vi "CenterFinder_6points_2points.vi"() -> ()   [LabVIEW 2016]
uses:
  Control/ProcessCtl.ctl
  <vilib>/userdefined/High Color/IMAQdx.ctl
  <vilib>/Utility/config.llb/Read Key (String).vi
  <vilib>/Utility/config.llb/Write Key (Double).vi
  <vilib>/vision/driver/NI_Vision_Acquisition_Software.lvlib
  <vilib>/vision/NI_Vision_Development_Module.lvlib
  <vilib>/Utility/config.llb/NI_LVConfig.lvlib
panel:
  out "output cluster":T1
  out "Array":T2(array[cluster])
  in  "stop 2":bool
  out "1":u32[](array[colorbox])
  in  "MoveTo":bool
  out "Boolean":bool=TRUE
  in  "GoToXY":bool
  out "Tip Center":cluster{"X":dbl, "Y":dbl, "Z":dbl}
  in  "Minimum Edge Strength":dbl=10.0
  out "Camera Center":cluster{"X":dbl, "Y":dbl, "Z":dbl}
  in  "Delete":bool caption="Retake"
  in  "Retake":bool caption="Delete"
  in  "Next":bool
  in  "Process":bool
  in  "Acquire":bool
  in  "stop":bool
  out "Image":T3(plugin-control)
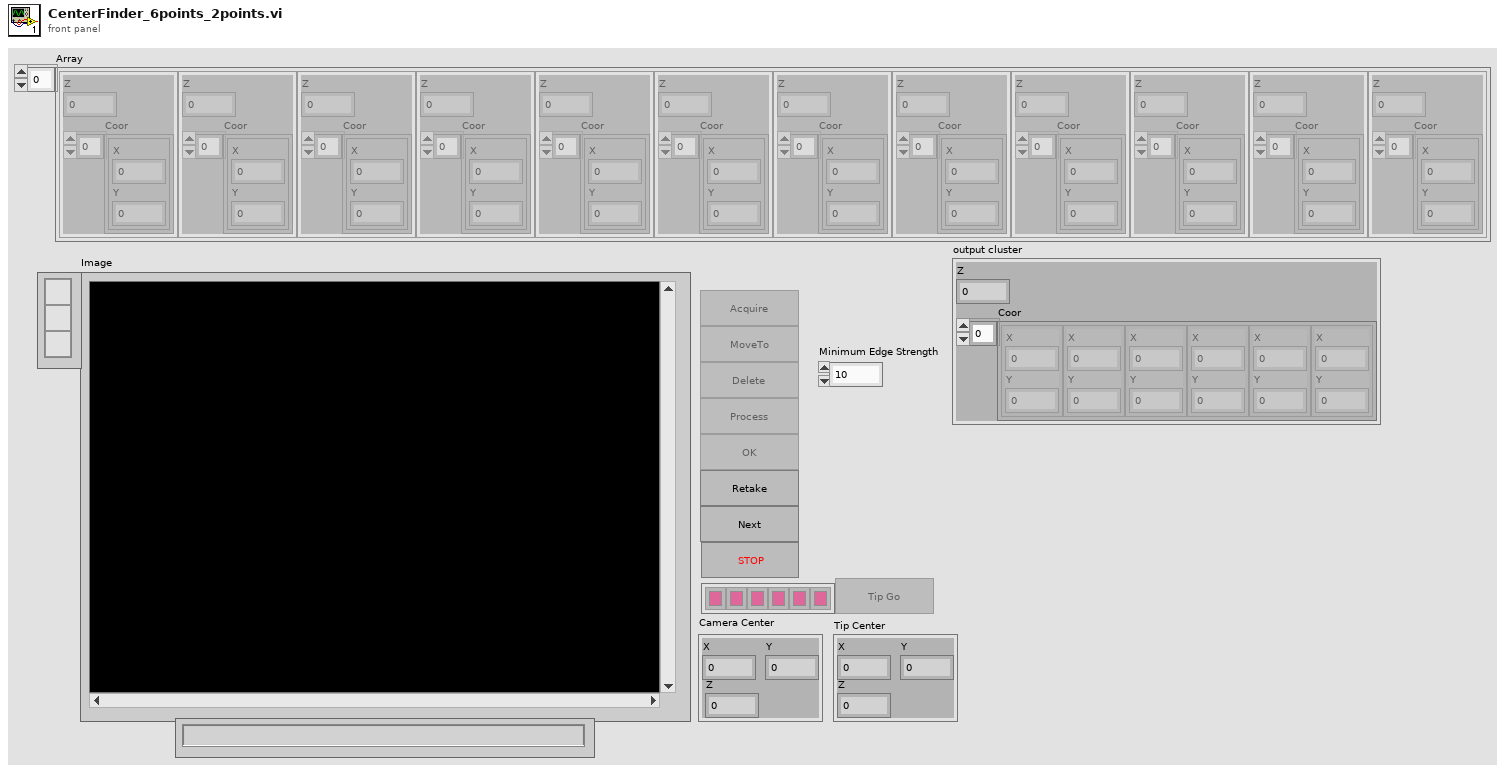
[diagram p1: front panel]
types:
  T1 = cluster{"Z":dbl, "Coor":cluster{"X":sgl, "Y":sgl}[]}
  T2 = cluster{"Z":dbl, "Coor":cluster{"X":sgl, "Y":sgl}[]}[]
  T3 = typedef "IMAQ Image.ctl" = refnum<image>
  T4 = cluster{"Line Segment":cluster{"Point 1":cluster{"X":sgl, "Y":sgl}, "Point 2":cluster{"X":sgl, "Y":sgl}}, "Z":dbl}[]
  T5 = typedef "IMAQdx.ctl" = refnum<k21>
  T6 = typedef "ProcessCtl.ctl" = enum16{"Idle", "Acquire", "Process", "Abort", "Initialize", "Wait"}
  T7 = typedef "NI_LVConfig.lvlib/Config Data RefNum.ctl" = refnum<k1>
  T8 = enum8{"Enabled", "Disabled", "Disabled and Grayed Out"}
  T9 = cluster{"Edge Polarity":u16, "Kernel Size":u32, "Width":u32, "Minimum Edge Strength":dbl, "Interpolation Type":u16, "Data Processing Method":u16}
  T10 = typedef "IMAQ Line" = cluster{"Start X":i32, "Start Y":i32, "End X":i32, "End Y":i32}
  T11 = typedef "Image Type" = u32
  T12 = typedef "ROI Descriptor" = cluster{"Global Rectangle":i32[], "Contours":cluster{"ID":enum32{"External", "Internal"}, "Type":u32, "Coordinates":i32[]}[]}
  T13 = cluster{"Global Rectangle":i32[], "Contours":cluster{"Contour Type":u32, "ROI Type":u32, "Points":i32[]}[]}
  T14 = typedef "Edge New.ctl" = cluster{"Location (Pixel)":cluster{"X":sgl, "Y":sgl}, "Location (Real-World)":cluster{"X":sgl, "Y":sgl}, "Distance (Pixel)":dbl, "Distance (Real-World)":dbl, "Strength":dbl, "Noise":dbl, "Rising?":bool}
  T15 = typedef "ControllerDiagPacket.ctl" = cluster{"Number of Diag Packets":i32, "Axes":T16[], "error":errorcluster}
  T16 = typedef "AxisDiagPacket.ctl" = cluster{"Axis Name":string, "Analog Input 0":dbl, "Analog Input 1":dbl, "Axis Fault (num)":i32, "Axis Fault (str)":string, "Axis Fault (bits)":cluster{"AmplifierFault":bool, "AmplifierTemperatureFault":bool, "CcwEndOfTravelLimitFault":bool, "CcwSoftwareLimitFault":bool, "CommunicationLostFault":bool, "CwEndOfTravelLimitFault":bool, "CwSoftwareLimitFault":bool, "EmergencyStopFault":bool, "EncoderFault":bool, "ExternalFault":bool, "FeedbackScalingFault":bool, "GantryMisalignFault ":bool, "HallSensorFault":bool, "InPositionTimeoutFault":bool, "InternalFault":bool, "MarkerSearchFault":bool, "MaxVelocityCommandFault":bool, "MissedInterruptFault":bool, "MotorTemperatureFault":bool, "None":bool, "OverCurrentFault":bool, "PositionErrorFault":bool, "PositionFeedbackFault":bool, "PowerSupplyFault":bool, "ProbeInputFault":bool, "SafeZoneFault":bool, "VelocityErrorFault":bool, "VelocityFeedbackFault":bool, "VoltageClampFault":bool}, "Axis Status (num)":i32, "Axis Status (str)":string, "Axis Status (bits)":cluster{"BacklashActive":bool, "CalibrationEnabled1D":bool, "CalibrationEnabled2D":bool, "CommandValid":bool, "DriveAbortPending":bool, "DrivePending":bool, "Enabling":bool, "GainMappingEnabled":bool, "GantryAligned":bool, "GantryRealigning":bool, "Homed":bool, "Homing":bool, "IFOVEnabled":bool, "JogGenerating":bool, "Jogging":bool, "JoystickControl":bool, "MasterSlaveControl":bool, "MotionBlocked":bool, "MotionClamped":bool, "MoveDone":bool, "None":bool, "NotVirtual":bool, "Profiling":bool, "Stability0":bool, "Stability1":bool, "TrajectoryFiltering":bool, "WaitDone":bool}, "Current Command":sgl, "Current Error":sgl, "Current Feedback":sgl, "Digital Inputs":i32, "Digital Outputs":i32, "Drive Status":i32, "Drive Status (str)":string, "Drive Status (bits)":cluster{"AccelerationPhase":bool, "AutofocusActive":bool, "BrakeOutput":bool, "CcwEndOfTravelLimitInput":bool, "CosineEncoderError":bool, "CurrentClamp":bool, "CwEndOfTravelLimitInput":bool, "DecelerationPhase":bool, "DualLoopActive":bool, "EmergencyStopInput":bool, "Enabled":bool, "EncoderClipping":bool, "GalvoCalibrationEnabled":bool, "GalvoPowerCorrection":bool, "HallAInput":bool, "HallBInput":bool, "HallCInput":bool, "HighResolutionMode":bool, "HomeLimitInput":bool, "InPosition":bool, "InPosition2":bool, "MarkerInput":bool, "MarkerLatch":bool, "MoveActive":bool, "NoMotorSupply":bool, "None":bool, "PowerLimiting":bool, "ProgrammingFlash":bool, "ProgrammingMXH":bool, "PSOHaltLatch":bool, "ServoControl":bool, "SineEncoderError":bool}, "Position Feedback Auxiliary":dbl, "Position Command":dbl, "Position Error":dbl, "Position Feedback":dbl, "Program Position Command":dbl, "Program Position Error":dbl, "Program Position Feedback":dbl, "Velocity Command":dbl, "Velocity Error":dbl, "Velocity Feedback":dbl}
  T17 = cluster{"Line Segment":cluster{"Point 1":cluster{"X":sgl, "Y":sgl}, "Point 2":cluster{"X":sgl, "Y":sgl}}, "Z":dbl}
  T18 = cluster{"Point 1":cluster{"X":sgl, "Y":sgl}, "Point 2":cluster{"X":sgl, "Y":sgl}}
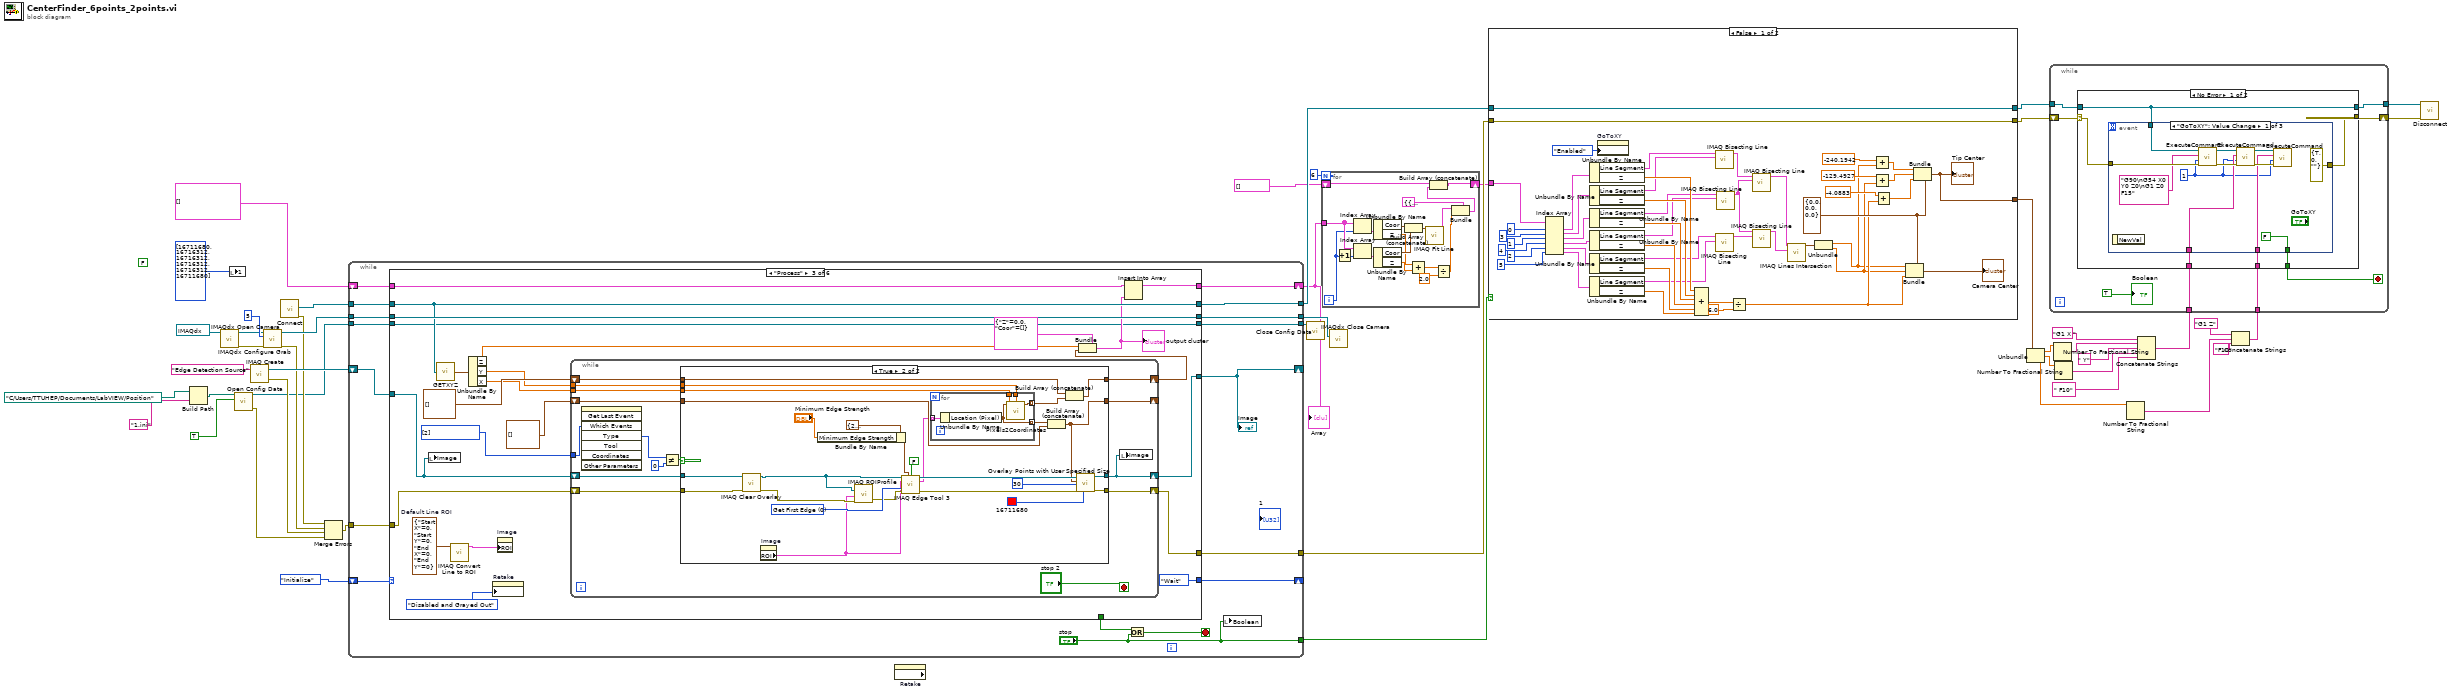
[diagram p0: block diagram]
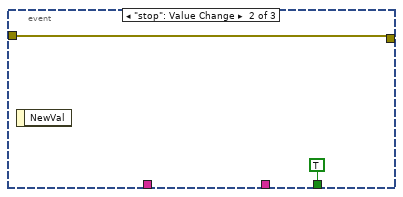
[diagram p2: hidden frame]
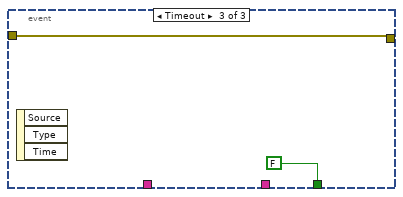
[diagram p3: hidden frame]
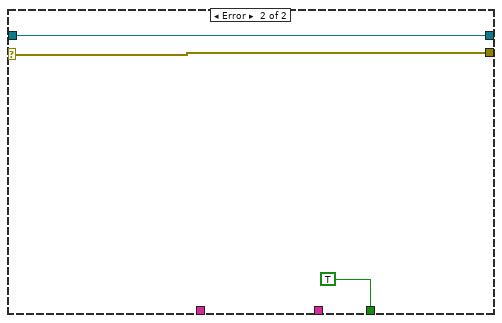
[diagram p4: hidden frame]
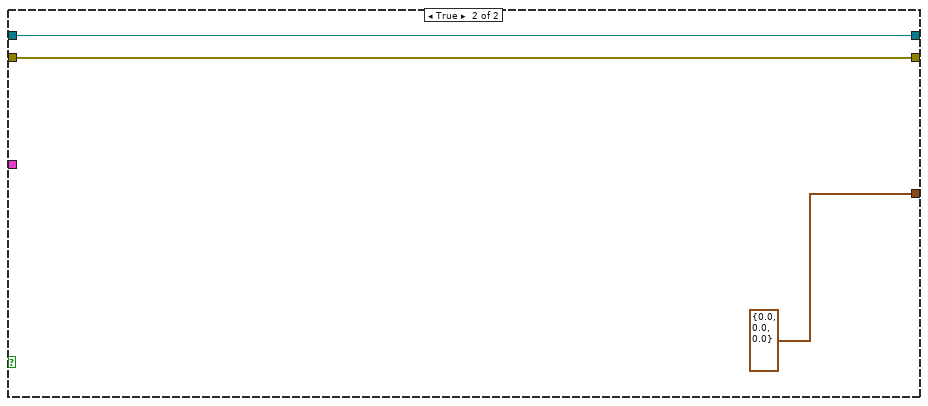
[diagram p5: hidden frame]
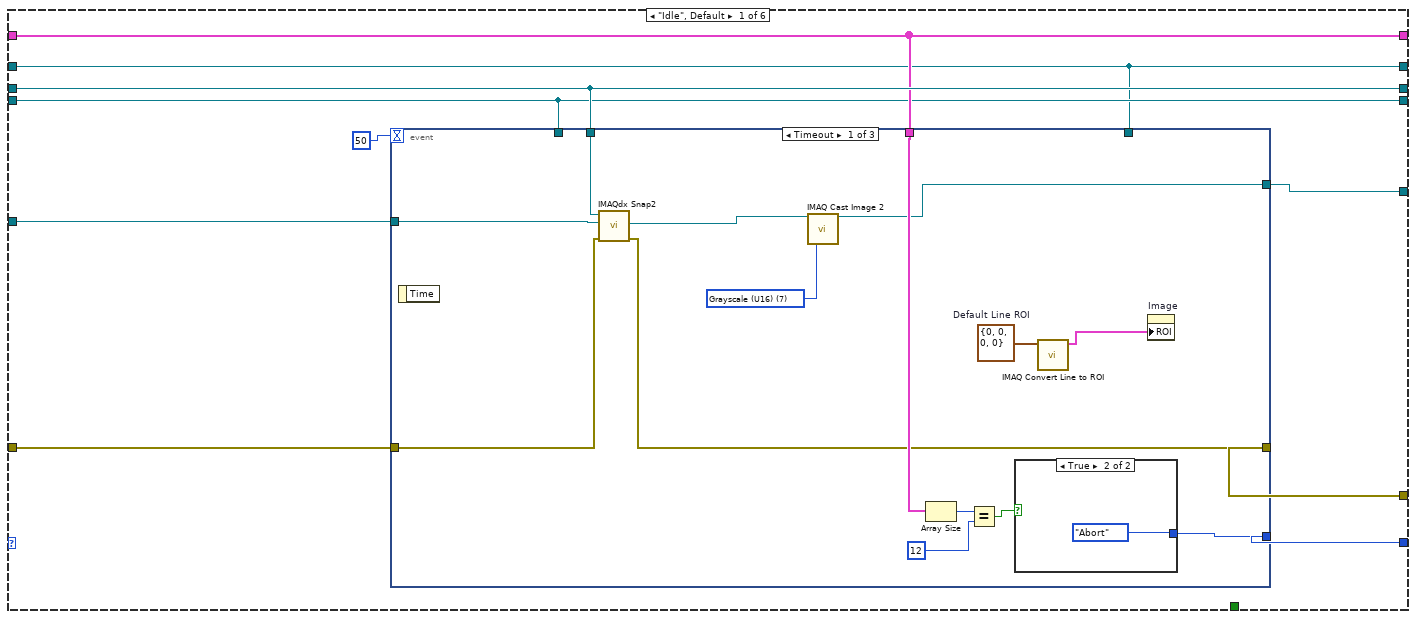
[diagram p6: hidden frame]
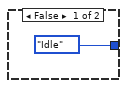
[diagram p7: hidden frame]
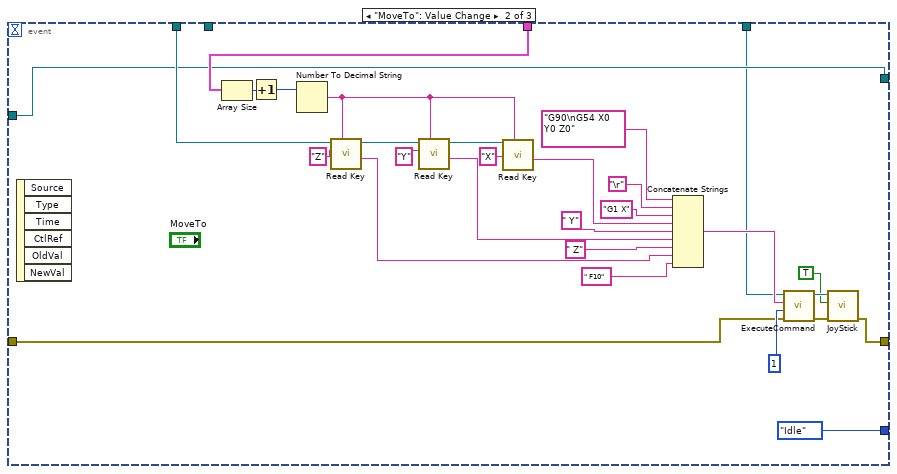
[diagram p8: hidden frame]
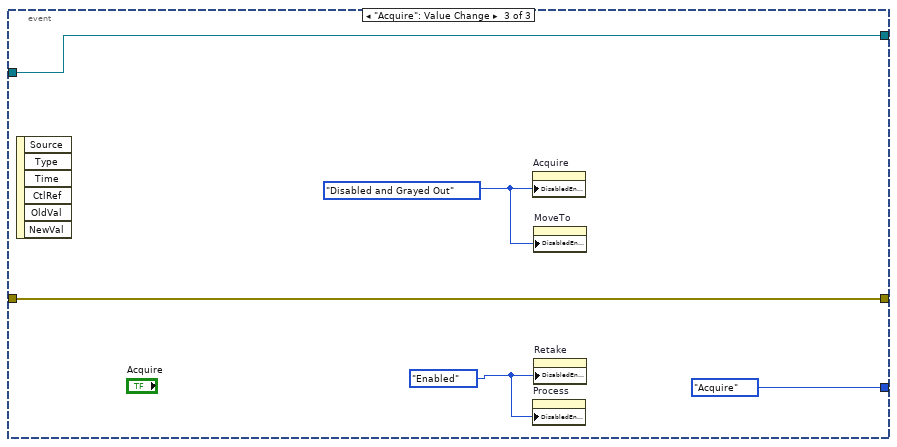
[diagram p9: hidden frame]
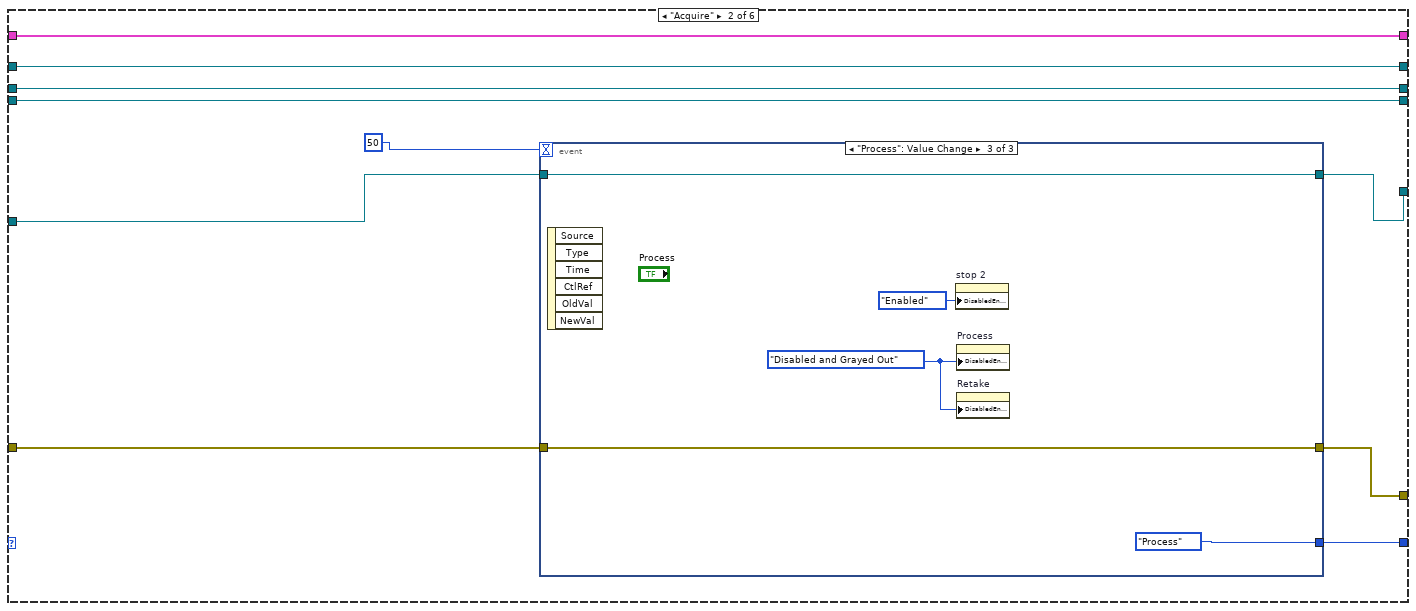
[diagram p10: hidden frame]
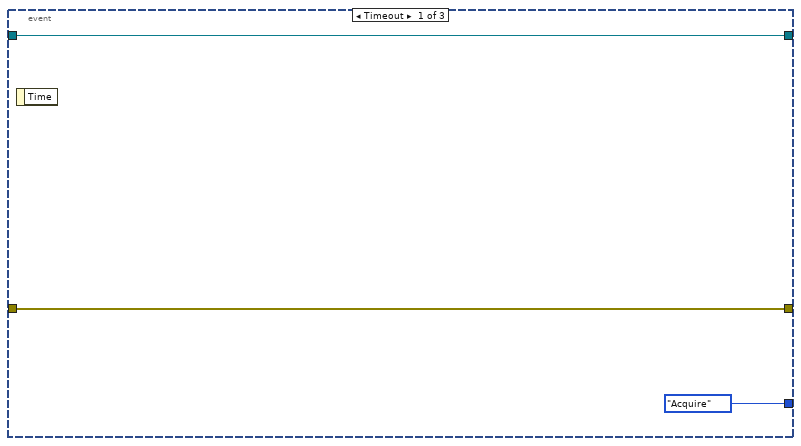
[diagram p11: hidden frame]
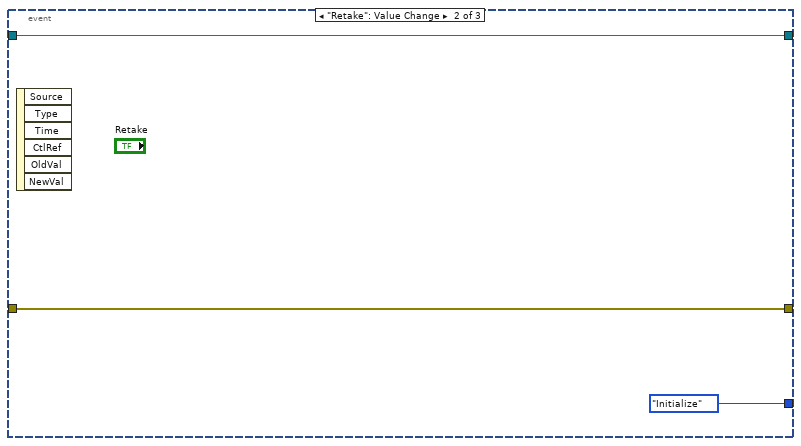
[diagram p12: hidden frame]
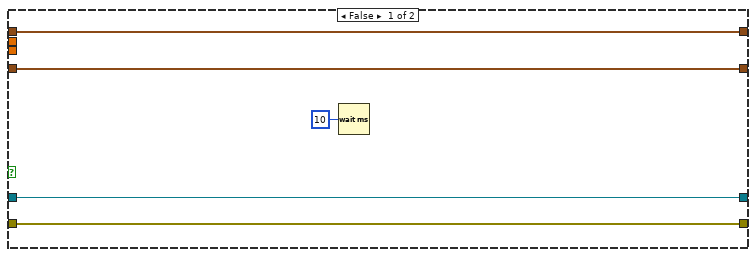
[diagram p13: hidden frame]
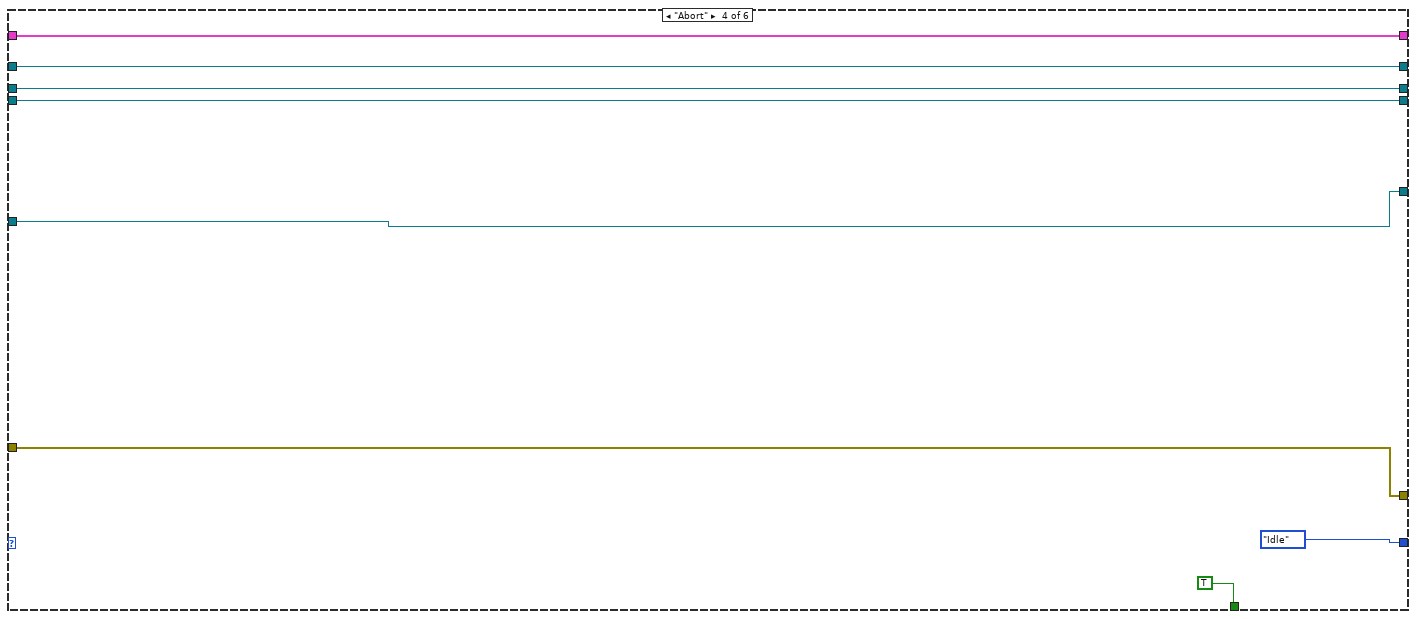
[diagram p14: hidden frame]
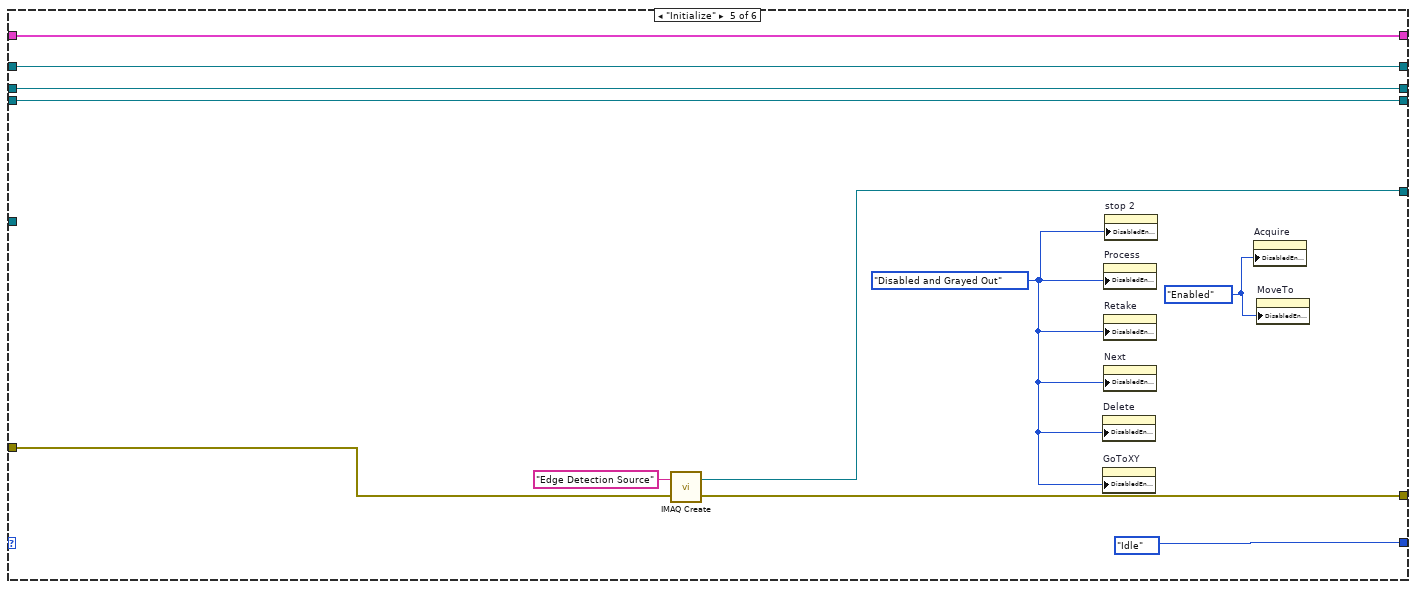
[diagram p15: hidden frame]
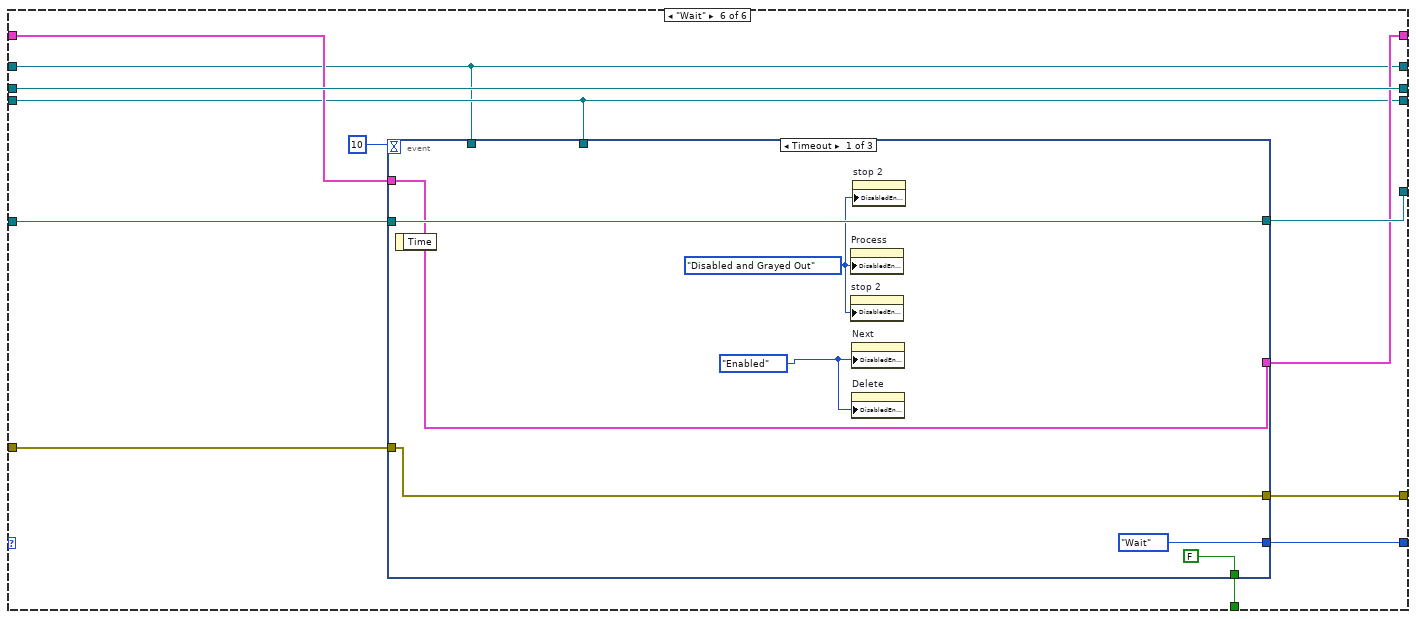
[diagram p16: hidden frame]
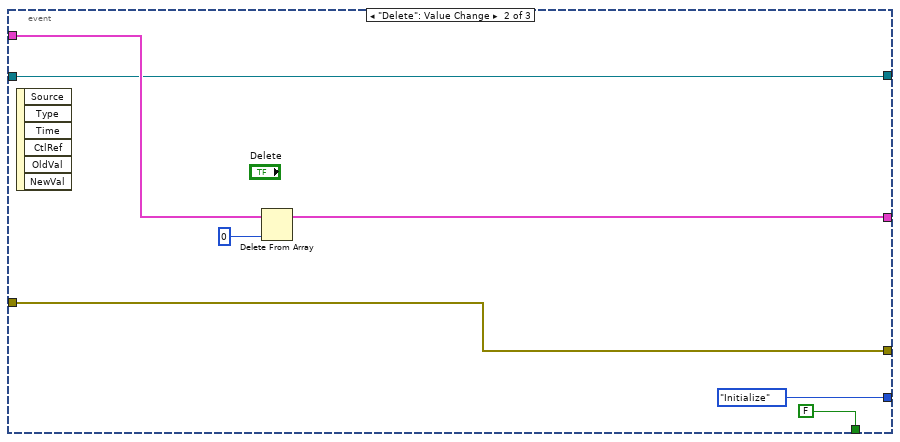
[diagram p17: hidden frame]
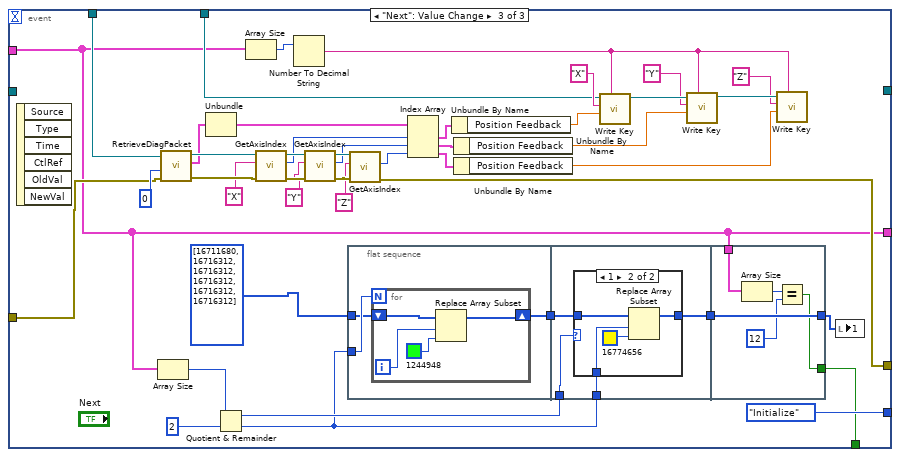
[diagram p18: hidden frame]
diagram:
  (unwired) FALSE ("1")
  n1 = Build Path(base path=path "C:/Users/TTUHEP/Documents/LabVIEW/Position", name or relative path="1.ini") -> (appended path=w14:path)
  n2 = call <vilib>:"IMAQdx Open Camera.vi"("Session In"=T5 "cam0") -> ("error out"=w47:errorcluster, "Session Out"=w1:T5)  [unwired: 9 in]
  n3 = local write "1"(u32[] [16711680, 16716312, 16716312, 16716312, 16716312, 16711680] ("1 2")) -> ()
  n4 = call <vilib>:"Open Config Data.vi"("create file if necessary (T)"=TRUE, "configuration file path"=w14) -> ("error out"=w13:errorcluster, "refnum"=w12:T7)  [unwired: 7 in, 1 out]
  n5 = call "IMAQ Create"("Image Name"="Edge Detection Source") -> ("New Image"=w45:T3, "error out"=w41:errorcluster)  [unwired: 4 in]
  n6 = call <vilib>:"IMAQdx Configure Grab.vi"("error in"=w47, "Number of Buffers"=u32 5, "Session In"=w1) -> ("error out"=w42:errorcluster, "Session Out"=w48:T5)  [unwired: 7 in]
  n7 = call "Connect.vi"() -> ("error out"=w23:errorcluster, "controller"=w24:refnum<k24>)  [unwired: 10 in]
  n8 = Merge Errors(w23, w42, w41, w13) -> (w40:errorcluster)
  n9 = while {
    tunnel: w48 -> [w56]
    tunnel: [w55] -> w43
    shift-right: [w62] -> _
    shift-left: w45 -> [w60]
    tunnel: w24 -> [w58]
    tunnel: [w57] -> w36
    tunnel: w40 -> [w65]
    shift-right: [w63] -> _
    shift-left: ProcessCtl."Initialize" -> [w64]
    tunnel: [w61] -> w37
    shift-right: [w52] -> w6
    shift-left: T2 [] -> [w59]
    tunnel: ["stop"] -> w38
    tunnel: w12 -> [w50]
    tunnel: [w49] -> w11
    stop <- w53 stop-if-true
    n10 = case shown="\"Process\"" w64 {
      tunnel: w65 -> [w75 w131 w168 w223 w236 w244]
      tunnel: [w72 w132 ProcessCtl."Wait" ProcessCtl."Idle" ProcessCtl."Idle" w249] -> w63
      tunnel: w60 -> [w74 w135 w156 w226 _ w251]
      tunnel: [w73 w134 w163 w226 w237 w250] -> w62
      tunnel: [w71 w130 w157 w223 w235 w245] -> w61
      tunnel: w59 -> [w69 w129 w159 w228 w234 w247]
      tunnel: [w69 w129 w158 w228 w234 w246] -> w52
      tunnel: w58 -> [w67 w128 w160 w222 w233 w241]
      tunnel: [w67 w128 w160 w222 w233 w241] -> w57
      tunnel: w56 -> [w70 w127 w161 w227 w232 w248]
      tunnel: [w70 w127 w161 w227 w232 w248] -> w55
      tunnel: [_ _ _ TRUE _ w240] -> w54
      tunnel: [w68 w126 w152 w221 w231 w242] -> w49
      tunnel: w50 -> [w68 w126 w152 w221 w231 w242]
      frame "Idle", Default {
        n11 = event shown="[0] Timeout" {
          selector: _ -> [_ _ _]
          dyn-events: _ -> [_ _ _]
          timeout: 50 -> [_ _ _]
          tunnel: w75 -> [w80 w93 w123]
          tunnel: w74 -> [w82 w98 w124]
          tunnel: w70 -> [w81 _ _]
          tunnel: [w83 w98 w124] -> w73
          tunnel: [w89 ProcessCtl."Idle" ProcessCtl."Acquire"] -> w72
          tunnel: [w79 w95 w123] -> w71
          tunnel: w69 -> [w88 w119 _]
          tunnel: w68 -> [_ w120 _]
          tunnel: w67 -> [_ w92 _]
          event Timeout {
            w77 = T10 {"Start X"=0, "Start Y"=0, "End X"=0, "End Y"=0}  # Default Line ROI
            w84 = T11 7 items=["Grayscale (U8)", "Grayscale (I16)", "Grayscale (SGL)", "Complex (CSG)", "RGB (U32)", "HSL (U32)", "RGB (U64)", "Grayscale (U16)"] ("Image Type")
            n12 = event-data() -> ()  [unwired: 1 in, 1 out]
            n13 = call <vilib>:"IMAQdx Snap2.vi"("error in"=w80, "Image In"=w82, "Session In"=w81) -> ("error out"=w79:errorcluster, "Image Out"=w78:T3)  [unwired: 6 in, 1 out]
            n14 = call "IMAQ Cast Image 2"("Image Src"=w78, "Image Type"=w84) -> ("Image Dst Out"=w83:T3)  [unwired: 12 in, 1 out]
            n15 = Array Size(array=w88) -> (size(s)=w87:i32)
            n16 = Equal?(x=w87, y=12) -> (x = y?=w85:bool)
            n17 = case shown="True" w85 {
              tunnel: [ProcessCtl."Idle" ProcessCtl."Abort"] -> w89
              frame False {
              }
              frame True {
              }
            }
            n18 = call "IMAQ Convert Line to ROI"("Line"=w77) -> ("ROI Descriptor"=w76:T12)  [unwired: 8 in, 1 out]
            n19 = property on="Image" class="ImageControl"("ROI"=w76) -> ()  [unwired: 2 in, 2 out]
          }
          event "MoveTo": Value Change {
            n20 = event-data() -> ()  [unwired: 1 in, 6 out]
            n21 = Array Size(array=w119) -> (size(s)=w118:i32)
            n22 = Increment(x=w118) -> (x+1=w100:i32)
            n23 = Number To Decimal String(number=w100) -> (decimal integer string=w117:string)  [unwired: 1 in]
            n24 = call-poly <vilib>:"Read Key.vi"("section"=w117, "key"="Z", "refnum"=w120) -> ("value"=w106:string, "refnum out"=w113:T7)  [unwired: 5 in, 2 out]
            n25 = call-poly <vilib>:"Read Key.vi"("section"=w117, "key"="Y", "refnum"=w113) -> ("value"=w107:string, "refnum out"=w112:T7)  [unwired: 5 in, 2 out]
            n26 = call-poly <vilib>:"Read Key.vi"("section"=w117, "key"="X", "refnum"=w112) -> ("value"=w108:string)  [unwired: 5 in, 3 out]
            n27 = Concatenate Strings("G90\nG54 X0 Y0 Z0", "\r", "G1 X", w108, " Y", w107, " Z", w106, " F10") -> (w102:string)
            n28 = call "ExecuteCommand.vi"("error in (no error)"=w93, "taskId"=1, "Command Code"=w102, "controller in"=w92) -> ("error out"=w96:errorcluster, "controller out"=w97:refnum<k24>)  [unwired: 5 in, 1 out]
            n29 = call "JoyStick.vi"("error in (no error)"=w96, "On/Off"=TRUE, ".NET Refnum in"=w97) -> ("error out"=w95:errorcluster)  [unwired: 7 in, 1 out]
          }
          event "Acquire": Value Change {
            w122 = T8."Enabled" ("Disabled")
            w121 = T8."Disabled and Grayed Out" ("Disabled")
            n30 = event-data() -> ()  [unwired: 1 in, 6 out]
            n31 = property on="Acquire" class="Bool"("DisabledEnum"=w121) -> ()  [unwired: 2 in, 2 out]
            n32 = property on="Process" class="Bool"("DisabledEnum"=w122) -> ()  [unwired: 2 in, 2 out]
            n33 = property on="MoveTo" class="Bool"("DisabledEnum"=w121) -> ()  [unwired: 2 in, 2 out]
            n34 = property on="Retake" class="Bool"("DisabledEnum"=w122) -> ()  [unwired: 2 in, 2 out]
          }
        }
      }
      frame "Acquire" {
        n35 = event shown="[2] \"Process\": Value Change" {
          selector: _ -> [_ _ _]
          dyn-events: _ -> [_ _ _]
          timeout: 50 -> [_ _ _]
          tunnel: w135 -> [w138 w139 w144]
          tunnel: [w138 w139 w144] -> w134
          tunnel: [ProcessCtl."Acquire" ProcessCtl."Initialize" ProcessCtl."Process"] -> w132
          tunnel: w131 -> [w136 w140 w145]
          tunnel: [w136 w140 w145] -> w130
          event Timeout {
            n36 = event-data() -> ()  [unwired: 1 in, 1 out]
          }
          event "Retake": Value Change {
            n37 = event-data() -> ()  [unwired: 1 in, 6 out]
          }
          event "Process": Value Change {
            w142 = T8."Disabled and Grayed Out" ("Disabled")
            n38 = event-data() -> ()  [unwired: 1 in, 6 out]
            n39 = property on="stop 2" class="Bool"("DisabledEnum"=T8."Enabled" ("Disabled")) -> ()  [unwired: 2 in, 2 out]
            n40 = property on="Process" class="Bool"("DisabledEnum"=w142) -> ()  [unwired: 2 in, 2 out]
            n41 = property on="Retake" class="Bool"("DisabledEnum"=w142) -> ()  [unwired: 2 in, 2 out]
          }
        }
      }
      frame "Process" {
        w151 = T10 {"Start X"=0, "Start Y"=0, "End X"=0, "End Y"=0}  # Default Line ROI
        w169 = i32[] [2] items=["No  event", "Click event", "Draw event", "Move event", "Size event", "Scroll event", "Activate event", "Close event", "Double click event"] ("Events list (all)")
        n42 = local write "Image"(w156) -> ()
        n43 = call "GETXYZ.vi"(".NET Refnum in"=w160) -> ("XYZ"=w166:cluster{"X":dbl, "Y":dbl, "Z":dbl})
        n44 = call "IMAQ Convert Line to ROI"("Line"=w151) -> ("ROI Descriptor"=w150:T12)  [unwired: 8 in, 1 out]
        n45 = Unbundle By Name(w166) -> ("Z"=w147:dbl, "Y"=w165:dbl, "X"=w164:dbl)
        n46 = property on="Retake" class="Bool"("DisabledEnum"=T8."Disabled and Grayed Out" ("Disabled")) -> ()  [unwired: 2 in, 2 out]
        n47 = property on="Image" class="ImageControl"("ROI"=w150) -> ()  [unwired: 2 in, 2 out]
        n48 = while {
          tunnel: w169 -> [w184]
          tunnel: w165 -> [w180]
          tunnel: w164 -> [w179]
          shift-right: [w178] -> w157
          shift-left: w168 -> [w183]
          shift-right: [w181] -> w148
          shift-left: cluster{"X":sgl, "Y":sgl}[] [] -> [w182]
          shift-right: [w170] -> w163
          shift-left: w156 -> [w177]
          shift-right: [w175] -> _
          shift-left: cluster{"X":sgl, "Y":sgl}[] [] -> [w176]
          stop <- "stop 2" stop-if-true
          n49 = invoke on="Image" class="ImageControl" method="Get Last Event"("Which Events"=w184) -> ("Type"=w173:i32)  [unwired: 7 in, 7 out]
          n50 = Not Equal?(x=w173, y=0) -> (x != y?=w172:bool)
          n51 = case shown="True" w172 {
            tunnel: w183 -> [w186 w215]
            tunnel: w182 -> [w189 w214]
            tunnel: [w189 w213] -> w181
            tunnel: w180 -> [_ w212]
            tunnel: w179 -> [_ w211]
            tunnel: [w187 w210] -> w170
            tunnel: [w186 w209] -> w178
            tunnel: w177 -> [w187 w208]
            tunnel: w176 -> [w188 w207]
            tunnel: [w188 w190] -> w175
            frame False {
              n52 = Wait (ms)(milliseconds to wait=u32 10) -> ()  [unwired: 1 out]
            }
            frame True {
              w206 = u16 0 items=["Get First Edge", "Get First + Last Edge", "Get All Edges", "Get Best Edge"] ("Process")
              n53 = call "IMAQ Clear Overlay"("error in (no error)"=w215, "Image"=w208) -> ("error out"=w197:errorcluster, "Image Out"=w196:T3)  [unwired: 8 in]
              n54 = property on="Image" class="ImageControl"() -> ("ROI"=w191:T13)  [unwired: 2 in, 2 out]
              n55 = Bundle By Name(cluster=T9 {"Edge Polarity"=2, "Kernel Size"=37, "Width"=5, "Minimum Edge Strength"=10.0, "Interpolation Type"=0, "Data Processing Method"=1} ("Edge Options"), "Minimum Edge Strength"="Minimum Edge Strength") -> (w193:T9)
              n56 = call "IMAQ ROIProfile"("error in (no error)"=w197, "ROI Descriptor"=w191, "Image"=w196) -> ("error out"=w198:errorcluster)  [unwired: 1 in, 4 out]
              n57 = call "IMAQ Edge Tool 3"("Image"=w196, "Edge Options"=w193, "Optimized Mode"=FALSE, "ROI Descriptor"=w191, "Process"=w206, "error in (no error)"=w198) -> ("Image (duplicate)"=w204:T3, "Edge Information"=w199:T14[], "error out"=w203:errorcluster)  [unwired: 5 in, 2 out]
              n58 = for {
                tunnel: w199 -> [w220] mode=indexing
                tunnel: [w219] -> w201 mode=indexing
                tunnel: w212 -> [w218]
                tunnel: w211 -> [w217]
                tunnel: [w216] -> w195 mode=indexing
                n59 = Unbundle By Name(w220) -> ("Location (Pixel)"=w216:cluster{"X":sgl, "Y":sgl})
                n60 = call "Pixels2Coordinates.vi"("Y"=w218, "X"=w217, "Location (Pixel)"=w216) -> ("output cluster"=w219:cluster{"X":sgl, "Y":sgl})  [unwired: 8 in]
              }
              n61 = Build Array (concatenate)(w195, w207) -> (w190:cluster{"X":sgl, "Y":sgl}[])
              n62 = Build Array (concatenate)(w214, w201) -> (w213:cluster{"X":sgl, "Y":sgl}[])
              n63 = call "Overlay Points with User Specified Size.vi"("Color"=u32 16711680, "error in"=w203, "Point Diameter (5)"=30, "Points"=w190, "Image In"=w204) -> ("error out"=w209:errorcluster, "Image Out"=w210:T3)  [unwired: 5 in]
            }
          }
          n64 = local write "Image"(w170) -> ()
        }
        n65 = Bundle(cluster=T1 {"Z"=0.0, "Coor"=[]}, "Z"=w147, "Coor"=w148) -> (w153:T1)
        "output cluster" <- w153
        n66 = Insert Into Array(array=w159, new element=w153) -> (w158:T2)  [unwired: 1 in]
      }
      frame "Abort" {
      }
      frame "Initialize" {
        w229 = T8."Disabled and Grayed Out" ("Disabled")
        w230 = T8."Enabled" ("Disabled")
        n67 = call "IMAQ Create"("Image Name"="Edge Detection Source", "error in (no error)"=w236) -> ("New Image"=w237:T3, "error out"=w235:errorcluster)  [unwired: 3 in]
        n68 = property on="Delete" class="Bool"("DisabledEnum"=w229) -> ()  [unwired: 2 in, 2 out]
        n69 = property on="GoToXY" class="Bool"("DisabledEnum"=w229) -> ()  [unwired: 2 in, 2 out]
        n70 = property on="Process" class="Bool"("DisabledEnum"=w229) -> ()  [unwired: 2 in, 2 out]
        n71 = property on="Retake" class="Bool"("DisabledEnum"=w229) -> ()  [unwired: 2 in, 2 out]
        n72 = property on="Next" class="Bool"("DisabledEnum"=w229) -> ()  [unwired: 2 in, 2 out]
        n73 = property on="stop 2" class="Bool"("DisabledEnum"=w229) -> ()  [unwired: 2 in, 2 out]
        n74 = property on="Acquire" class="Bool"("DisabledEnum"=w230) -> ()  [unwired: 2 in, 2 out]
        n75 = property on="MoveTo" class="Bool"("DisabledEnum"=w230) -> ()  [unwired: 2 in, 2 out]
      }
      frame "Wait" {
        n76 = event shown="[0] Timeout" {
          selector: _ -> [_ _ _]
          dyn-events: _ -> [_ _ _]
          timeout: 10 -> [_ _ _]
          tunnel: w251 -> [w258 w262 _]
          tunnel: [w258 w262 _] -> w250
          tunnel: [ProcessCtl."Wait" ProcessCtl."Initialize" ProcessCtl."Initialize"] -> w249
          tunnel: w247 -> [w256 w265 w267]
          tunnel: [w256 w264 w267] -> w246
          tunnel: [w255 w260 w290] -> w245
          tunnel: w244 -> [w255 w260 w276]
          tunnel: w242 -> [_ _ w300]
          tunnel: w241 -> [_ _ w277]
          tunnel: [FALSE FALSE w266] -> w240
          event Timeout {
            w254 = T8."Enabled" ("Disabled")
            w253 = T8."Disabled and Grayed Out" ("Disabled")
            n77 = event-data() -> ()  [unwired: 1 in, 1 out]
            n78 = property on="Process" class="Bool"("DisabledEnum"=w253) -> ()  [unwired: 2 in, 2 out]
            n79 = property on="stop 2" class="Bool"("DisabledEnum"=w253) -> ()  [unwired: 2 in, 2 out]
            n80 = property on="Next" class="Bool"("DisabledEnum"=w254) -> ()  [unwired: 2 in, 2 out]
            n81 = property on="Delete" class="Bool"("DisabledEnum"=w254) -> ()  [unwired: 2 in, 2 out]
            n82 = property on="stop 2" class="Bool"("DisabledEnum"=w253) -> ()  [unwired: 2 in, 2 out]
          }
          event "Delete": Value Change {
            n83 = event-data() -> ()  [unwired: 1 in, 6 out]
            n84 = Delete From Array(array=w265, index=0) -> (array with subset deleted=w264:T2)  [unwired: 1 in, 1 out]
          }
          event "Next": Value Change {
            n85 = event-data() -> ()  [unwired: 1 in, 6 out]
            n86 = Array Size(array=w267) -> (size(s)=w275:i32)
            n87 = call "RetrieveDiagPacket.vi"("error in (no error)"=w276, "axisMask"=0, "Controller In"=w277) -> ("error out"=w293:errorcluster, "ControllerDiagPacket"=w296:T15, "Controller Out"=w299:refnum<k24>)  [unwired: 6 in]
            n88 = Unbundle(w296) -> ("Axes"=w295:T16[])  [unwired: 2 out]
            n89 = Quotient & Remainder(x=w275, y=2) -> (x-y*floor(x/y)=w272:i32, floor(x/y)=w271:i32)
            n90 = Array Size(array=w267) -> (size(s)=w307:i32)
            n91 = call "GetAxisIndex.vi"("error in (no error)"=w293, "axis name"="X", "controller in"=w299) -> ("error out"=w292:errorcluster, "axis index"=w287:i32, "controller out"=w298:refnum<k24>)  [unwired: 6 in]
            n92 = Number To Decimal String(number=w307) -> (decimal integer string=w306:string)  [unwired: 1 in]
            n93 = call "GetAxisIndex.vi"("error in (no error)"=w292, "axis name"="Y", "controller in"=w298) -> ("error out"=w291:errorcluster, "axis index"=w288:i32, "controller out"=w297:refnum<k24>)  [unwired: 6 in]
            n94 = flat-sequence {
              tunnel: w271 -> [w311]
              tunnel: u32[] [16711680, 16716312, 16716312, 16716312, 16716312, 16716312] ("1 2") -> [w310]
              tunnel: [w309] -> w273
              tunnel: w273 -> [w318]
              tunnel: w272 -> [w319]
              tunnel: w271 -> [w317]
              tunnel: [w316] -> w268
              tunnel: [w329] -> w269
              tunnel: w268 -> [w329]
              tunnel: w267 -> [w328]
              tunnel: [w325] -> w266
              frame #0 {
                n95 = for {
                  N: w311 -> [_]
                  shift-right: [w313] -> w309
                  shift-left: w310 -> [w315]
                  i -> [w314]
                  n96 = Replace Array Subset(array=w315, new element=u32 1244948 ("LED"), index=w314) -> (w313:u32[])
                }
              }
              frame #1 {
                n97 = case shown="1" w319 {
                  tunnel: w318 -> [w320 w323]
                  tunnel: w317 -> [_ w324]
                  tunnel: [w320 w322] -> w316
                  frame 0, Default {
                  }
                  frame 1 {
                    n98 = Replace Array Subset(array=w323, new element=u32 16774656 ("LED"), index=w324) -> (w322:u32[])
                  }
                }
              }
              frame #2 {
                n99 = Array Size(array=w328) -> (size(s)=w327:i32)
                n100 = Equal?(x=w327, y=12) -> (x = y?=w325:bool)
              }
            }
            n101 = call "GetAxisIndex.vi"("error in (no error)"=w291, "axis name"="Z", "controller in"=w297) -> ("error out"=w290:errorcluster, "axis index"=w289:i32)  [unwired: 6 in, 1 out]
            n102 = Index Array(array=w295, index #1=w287, index #2=w288, index #3=w289) -> (element #1=w286:T16, element #2=w285:T16, element #3=w284:T16)
            n103 = Unbundle By Name(w286) -> ("Position Feedback"=w283:dbl)
            n104 = Unbundle By Name(w285) -> ("Position Feedback"=w282:dbl)
            n105 = Unbundle By Name(w284) -> ("Position Feedback"=w281:dbl)
            n106 = call-poly <vilib>:"Write Key.vi"("section"=w306, "value"=w283, "key"="X", "refnum"=w300) -> ("refnum out"=w305:T7)  [unwired: 5 in, 2 out]
            n107 = call-poly <vilib>:"Write Key.vi"("section"=w306, "value"=w282, "key"="Y", "refnum"=w305) -> ("refnum out"=w304:T7)  [unwired: 5 in, 2 out]
            n108 = call-poly <vilib>:"Write Key.vi"("section"=w306, "value"=w281, "key"="Z", "refnum"=w304) -> ()  [unwired: 5 in, 3 out]
            n109 = local write "1"(w269) -> ()
          }
        }
      }
    }
    "Image" <- w62
    n110 = Or(x=w54, y="stop") -> (x .or. y?=w53:bool)
    n111 = local write "Boolean"("stop") -> ()
  }
  "Array" <- w6
  n112 = property on="Retake" class="Bool" props=["DisabledEnum"]() -> ()  [unwired: 2 in, 3 out]
  n113 = call <vilib>:"Close Config Data.vi"("refnum"=w11) -> ()  [unwired: 9 in, 2 out]
  n114 = for {
    N: 6 -> [_]
    tunnel: w6 -> [w346]
    shift-right: [w331] -> w3
    shift-left: T4 [] -> [w330]
    i -> [w337]
    n115 = Increment(x=w337) -> (x+1=w347:i32)
    n116 = Index Array(array=w346, index=w337) -> (element=w345:T1)
    n117 = Index Array(array=w346, index=w347) -> (element=w344:T1)
    n118 = Unbundle By Name(w345) -> ("Coor"=w342:cluster{"X":sgl, "Y":sgl}[], "Z"=w340:dbl)
    n119 = Unbundle By Name(w344) -> ("Coor"=w341:cluster{"X":sgl, "Y":sgl}[], "Z"=w339:dbl)
    n120 = Build Array (concatenate)(w342, w341) -> (w343:cluster{"X":sgl, "Y":sgl}[])
    n121 = Add(x=w340, y=w339) -> (x+y=w338:dbl)
    n122 = call "IMAQ Fit Line"("Points"=w343) -> ("Line Segment"=w335:T18)  [unwired: 5 in, 5 out]
    n123 = Divide(x=w338, y=2.0) -> (x/y=w336:dbl)
    n124 = Bundle(cluster=T17 {"Line Segment"={"Point 1"={"X"=0.0, "Y"=0.0}, "Point 2"={"X"=0.0, "Y"=0.0}}, "Z"=0.0}, "Line Segment"=w335, "Z"=w336) -> (w332:T17)
    n125 = Build Array (concatenate)(w330, w332) -> (w331:T4)
  }
  n126 = call <vilib>:"IMAQdx Close Camera.vi"("Session In"=w43) -> ()  [unwired: 10 in, 1 out]
  n127 = case shown="False" w38 {
    tunnel: w3 -> [w395 _]
    tunnel: w37 -> [w362 w397]
    tunnel: w36 -> [w348 w398]
    tunnel: [w348 w398] -> w34
    tunnel: [w362 w397] -> w35
    tunnel: [w353 cluster{"X":dbl, "Y":dbl, "Z":dbl} {"X"=0.0, "Y"=0.0, "Z"=0.0}] -> w33
    frame False {
      w360 = cluster{"X":dbl, "Y":dbl, "Z":dbl} {"X"=0.0, "Y"=0.0, "Z"=0.0}
      n128 = Index Array(array=w395, index #1=0, index #2=3, index #3=1, index #4=4, index #5=2, index #6=5) -> (element #1=w391:T17, element #2=w390:T17, element #3=w389:T17, element #4=w382:T17, element #5=w381:T17, element #6=w363:T17)
      n129 = Unbundle By Name(w391) -> ("Line Segment"=w374:T18, "Z"=w380:dbl)
      n130 = Unbundle By Name(w390) -> ("Line Segment"=w373:T18, "Z"=w379:dbl)
      n131 = Unbundle By Name(w389) -> ("Line Segment"=w372:T18, "Z"=w378:dbl)
      n132 = Unbundle By Name(w382) -> ("Line Segment"=w371:T18, "Z"=w377:dbl)
      n133 = Unbundle By Name(w381) -> ("Line Segment"=w370:T18, "Z"=w376:dbl)
      n134 = Unbundle By Name(w363) -> ("Line Segment"=w369:T18, "Z"=w375:dbl)
      n135 = property on="GoToXY" class="Bool"("DisabledEnum"=T8."Enabled" ("Disabled")) -> ()  [unwired: 2 in, 2 out]
      n136 = Compound Arithmetic op=ADD(w380, w379, w378, w377, w376, w375) -> (w388:dbl)
      n137 = call "IMAQ Bisecting Line"("Line 2"=w373, "Line 1"=w374) -> ("Bisecting Line"=w368:T18)  [unwired: 8 in, 1 out]
      n138 = call "IMAQ Bisecting Line"("Line 2"=w369, "Line 1"=w370) -> ("Bisecting Line"=w366:T18)  [unwired: 8 in, 1 out]
      n139 = call "IMAQ Bisecting Line"("Line 2"=w371, "Line 1"=w372) -> ("Bisecting Line"=w367:T18)  [unwired: 8 in, 1 out]
      n140 = Divide(x=w388, y=6.0) -> (x/y=w352:dbl)
      n141 = call "IMAQ Bisecting Line"("Line 2"=w367, "Line 1"=w368) -> ("Bisecting Line"=w365:T18)  [unwired: 8 in, 1 out]
      n142 = call "IMAQ Bisecting Line"("Line 2"=w366, "Line 1"=w367) -> ("Bisecting Line"=w364:T18)  [unwired: 8 in, 1 out]
      n143 = call "IMAQ Lines Intersection"("Line 2"=w364, "Line 1"=w365) -> ("Intersection Point"=w386:cluster{"X":sgl, "Y":sgl})  [unwired: 7 in, 2 out]
      n144 = Unbundle(w386) -> ("X"=w350:sgl, "Y"=w351:sgl)
      n145 = Add(x=-240.1942, y=w350) -> (x+y=w356:dbl)
      n146 = Add(x=-129.4927, y=w351) -> (x+y=w355:dbl)
      n147 = Add(x=-4.0883, y=w352) -> (x+y=w354:dbl)
      n148 = Bundle(cluster=w360, "X"=w350, "Y"=w351, "Z"=w352) -> (→"Camera Center":cluster{"X":dbl, "Y":dbl, "Z":dbl})
      n149 = Bundle(cluster=w360, "X"=w356, "Y"=w355, "Z"=w354) -> (w353:cluster{"X":dbl, "Y":dbl, "Z":dbl})
      "Tip Center" <- w353
    }
    frame True {
    }
  }
  n150 = Unbundle(w33) -> ("X"=w32:dbl, "Y"=w31:dbl, "Z"=w21:dbl)
  n151 = Number To Fractional String(number=w32) -> (F-format string=w29:string)  [unwired: 3 in]
  n152 = Number To Fractional String(number=w31) -> (F-format string=w27:string)  [unwired: 3 in]
  n153 = Number To Fractional String(number=w21) -> (F-format string=w20:string)  [unwired: 3 in]
  n154 = Concatenate Strings("G1 X ", w29, " Y", w27, " F10") -> (w25:string)
  n155 = Concatenate Strings("G1 Z", w20, "F10") -> (w18:string)
  n156 = while {
    shift-right: [w403] -> w9
    shift-left: w35 -> [w406]
    tunnel: w25 -> [w401]
    tunnel: w34 -> [w405]
    tunnel: [w404] -> w10
    tunnel: w18 -> [w399]
    stop <- w402 stop-if-true
    n157 = case shown="No Error" w406 {
      selector: w406 -> [w412 w430]
      tunnel: w405 -> [w411 w431]
      tunnel: [w411 w431] -> w404
      tunnel: [w409 w430] -> w403
      tunnel: [w410 TRUE] -> w402
      tunnel: w401 -> [w408 _]
      tunnel: w399 -> [w407 _]
      frame No Error {
        n158 = event shown="[0] \"GoToXY\": Value Change" {
          selector: _ -> [_ _ _]
          dyn-events: _ -> [_ _ _]
          timeout: _ -> [_ _ _]
          tunnel: w412 -> [w424 w425 w428]
          tunnel: w411 -> [w422 _ _]
          tunnel: [FALSE TRUE FALSE] -> w410
          tunnel: [errorcluster {"status"=TRUE, "code"=0, "source"=""} ("error IO") w425 w428] -> w409
          tunnel: w408 -> [w418 _ _]
          tunnel: w407 -> [w414 _ _]
          event "GoToXY": Value Change {
            w413 = 1
            n159 = event-data() -> ()  [unwired: 1 in, 1 out]
            n160 = call "ExecuteCommand.vi"("error in (no error)"=w424, "taskId"=w413, "Command Code"="G90\nG54 X0 Y0 Z0\nG1 Z0 F15", "controller in"=w422) -> ("error out"=w419:errorcluster, "controller out"=w423:refnum<k24>)  [unwired: 5 in, 1 out]
            n161 = call "ExecuteCommand.vi"("error in (no error)"=w419, "taskId"=w413, "Command Code"=w418, "controller in"=w423) -> ("error out"=w415:errorcluster, "controller out"=w416:refnum<k24>)  [unwired: 5 in, 1 out]
            n162 = call "ExecuteCommand.vi"("error in (no error)"=w415, "taskId"=w413, "Command Code"=w414, "controller in"=w416) -> ()  [unwired: 5 in, 3 out]
          }
          event "stop": Value Change {
            n163 = event-data() -> ()  [unwired: 1 in, 1 out]
          }
          event Timeout {
            n164 = event-data() -> ()  [unwired: 1 in, 3 out]
          }
        }
      }
      frame Error {
      }
    }
    "Boolean" <- TRUE
  }
  n165 = call "Disconnect.vi"("error in (no error)"=w9, "controller"=w10) -> ()  [unwired: 9 in, 1 out]
